vi "Position To Right of Previous Button.vi"(8 "error in (no error)":errorcluster, 10 "PreviousButton Ref":refnum<vi>, 11 "Button Ref":refnum<vi>) -> (0 "error out":errorcluster)   [LabVIEW 2014]
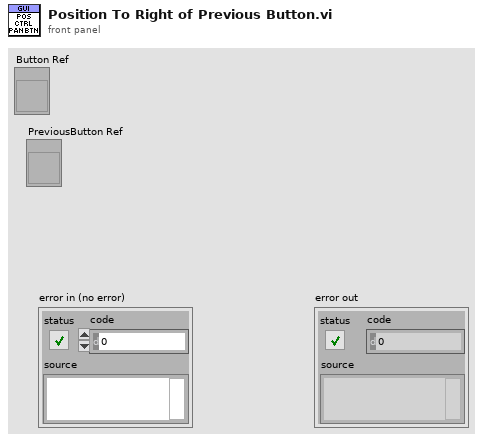
[diagram p1: front panel]
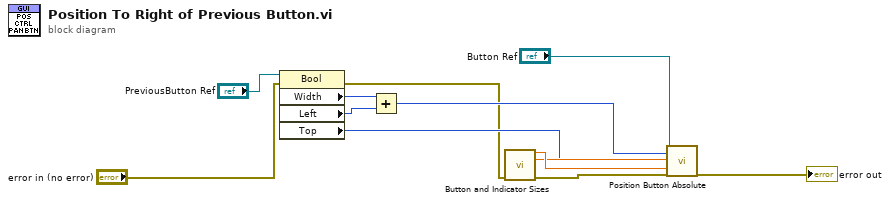
[diagram p0: block diagram]
diagram:
  n1 = property class="Bool"(reference="PreviousButton Ref", error in="error in (no error)") -> (error out=w1:errorcluster, "Width"=w6:u32, "Left"=w5:i32, "Top"=w4:i32)  [unwired: 1 out]
  n2 = Add(x=w6, y=w5) -> (x+y=w3:u32)
  n3 = call "Button and Indicator Sizes.vi"("error in (no error)"=w1) -> ("Button Width"=w9:dbl, "Button Height"=w8:dbl, "error out"=w10:errorcluster)  [unwired: 10 in, 2 out]
  n4 = call "Position Button Absolute.vi"("Button Ref"="Button Ref", "Left Offset (px)"=w3, "Top Offste (px)"=w4, "Height (px)"=w8, "Width (px)"=w9, "Error In"=w10) -> ("Error Out"=→"error out":errorcluster)  [unwired: 13 in]
